vi "OM Setup Page Filter.vi"(8 "OM Setup Page":T3, 9 "Rigid Connection In":bool, 10 "Number of\nLBCBs In":T2, 11 "LBCB Number In":T1) -> (3 "LBCB Number Out":T1)   [LabVIEW 2013]
uses:
  OM Setup Page.ctl
  Application/Number Of LBCBs.ctl
  Metadata/LBCB Number.ctl
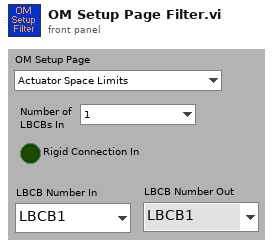
[diagram p1: front panel]
types:
  T1 = typedef "LBCB Number.ctl" = enum16{"LBCB1", "LBCB2"}
  T2 = typedef "Number Of LBCBs.ctl" = enum16{"1", "2"}
  T3 = typedef "OM Setup Page.ctl" = enum16{"Actuator Space Limits", "Cartesian Space Limits", "Autobalance & PID", "Timing and Logging", "LBCB Position", "Mixed Mode", "Calibration", "Channel Names", "External Sensors"}
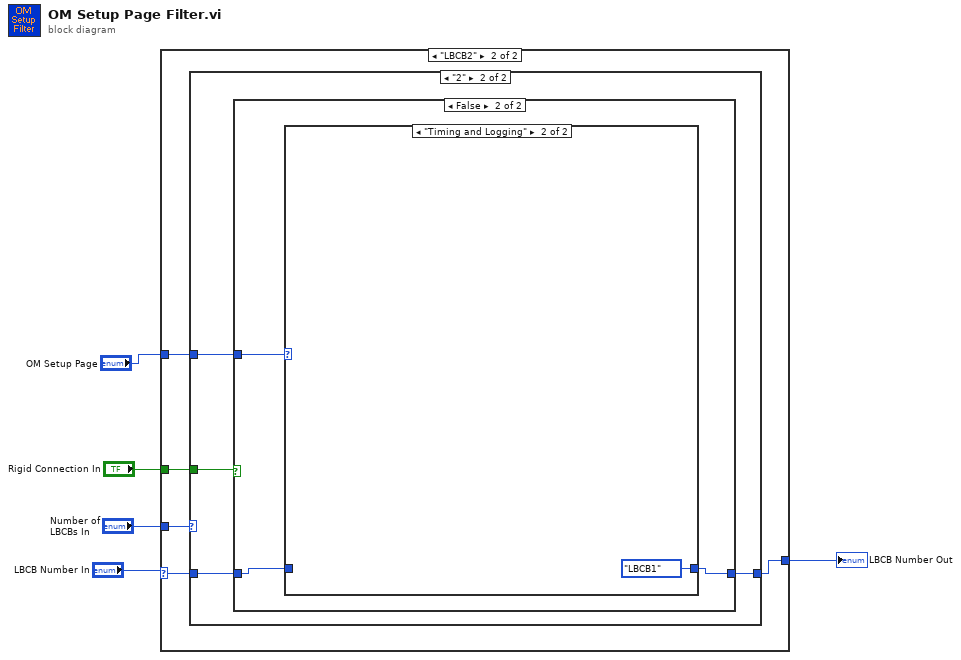
[diagram p0: block diagram]
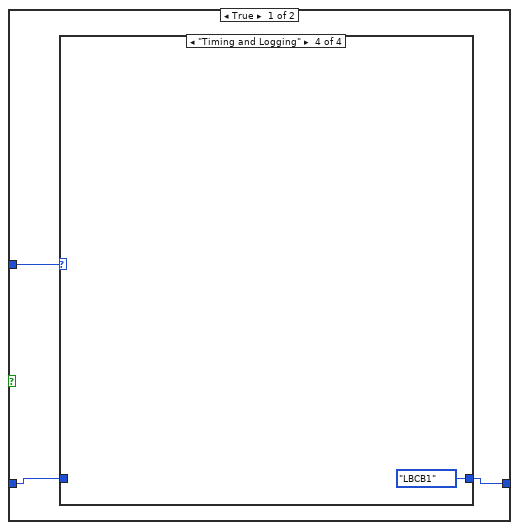
[diagram p4: hidden frame]
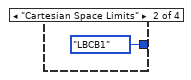
[diagram p6: hidden frame]
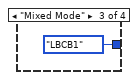
[diagram p7: hidden frame]
diagram:
  n1 = case shown="\"LBCB2\"" "LBCB Number In" {
    selector: "LBCB Number In" -> [w6 w10]
    tunnel: [w6 w9] -> w4
    tunnel: "Number of\nLBCBs In" -> [_ w11]
    tunnel: "Rigid Connection In" -> [_ w8]
    tunnel: "OM Setup Page" -> [_ w7]
    frame "LBCB1", Default {
    }
    frame "LBCB2" {
      n2 = case shown="\"2\"" w11 {
        tunnel: [w12 w14] -> w9
        tunnel: w10 -> [w12 w15]
        tunnel: w8 -> [_ w16]
        tunnel: w7 -> [_ w13]
        frame "1", Default {
        }
        frame "2" {
          n3 = case shown="False" w16 {
            tunnel: [w17 w24] -> w14
            tunnel: w15 -> [w18 w25]
            tunnel: w13 -> [w19 w26]
            frame True {
              n4 = case shown="\"Timing and Logging\"" w19 {
                tunnel: [w20 LBCB_Number."LBCB1" ("LBCB Number In") LBCB_Number."LBCB1" ("LBCB Number In") LBCB_Number."LBCB1" ("LBCB Number In")] -> w17
                tunnel: w18 -> [w20 _ _ _]
                frame "Actuator Space Limits", Default {
                }
                frame "Cartesian Space Limits" {
                }
                frame "Mixed Mode" {
                }
                frame "Timing and Logging" {
                }
              }
            }
            frame False {
              n5 = case shown="\"Timing and Logging\"" w26 {
                tunnel: [w27 LBCB_Number."LBCB1" ("LBCB Number In")] -> w24
                tunnel: w25 -> [w27 _]
                frame "Actuator Space Limits", Default {
                }
                frame "Timing and Logging" {
                }
              }
            }
          }
        }
      }
    }
  }
  "LBCB Number Out" <- w4
